vi "Guaman_Estrada_lv_DB_1_II_parcial.vi"() -> ()   [LabVIEW 2014]
panel:
  out "Array":bool[](array[boolean])
  in  "milliseconds to wait 2":u32
  in  "Boolean":bool
  in  "stop":bool
  in  "milliseconds to wait":u32
  out "led 8":bool
  out "led 7":bool
  out "led 6":bool
  out "led 5":bool
  out "led 4":bool
  out "led 3":bool
  out "led_ 2":bool
  out "led_1":bool
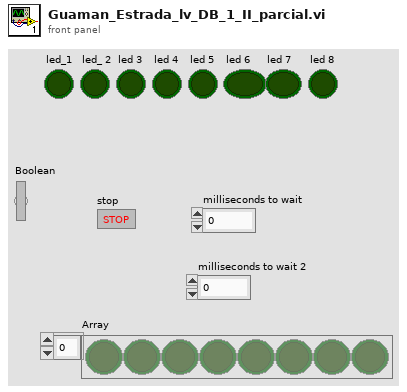
[diagram p1: front panel]
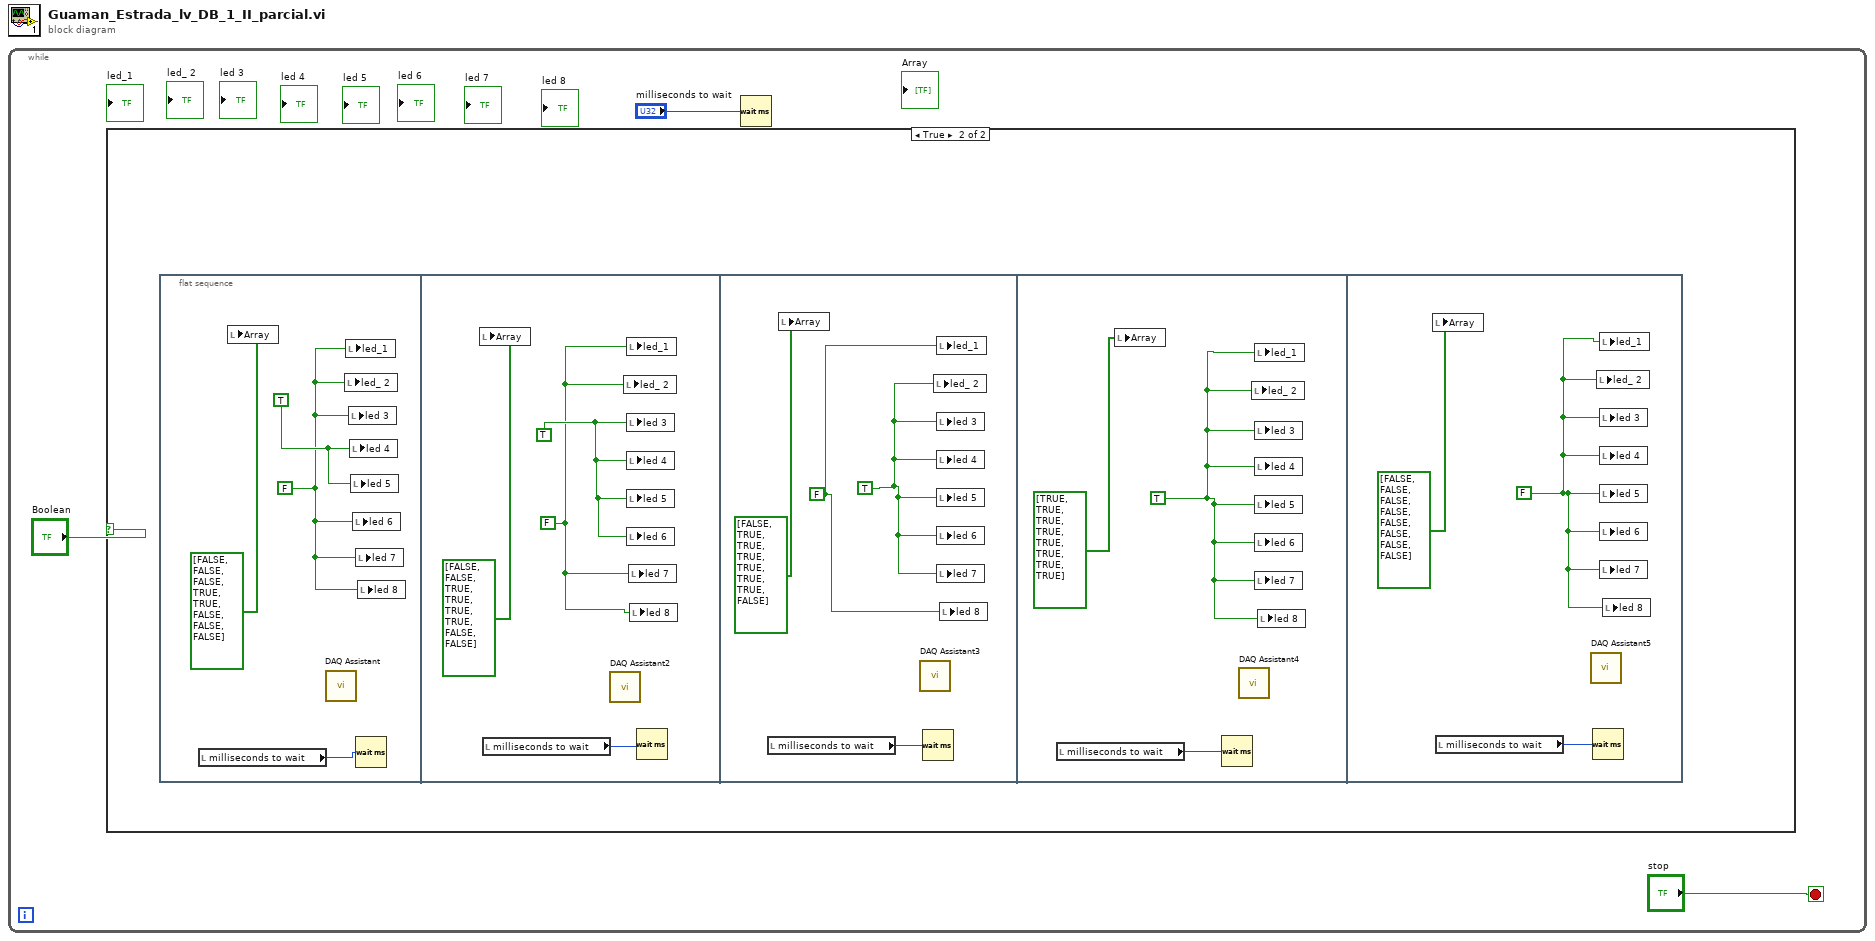
[diagram p0: block diagram]
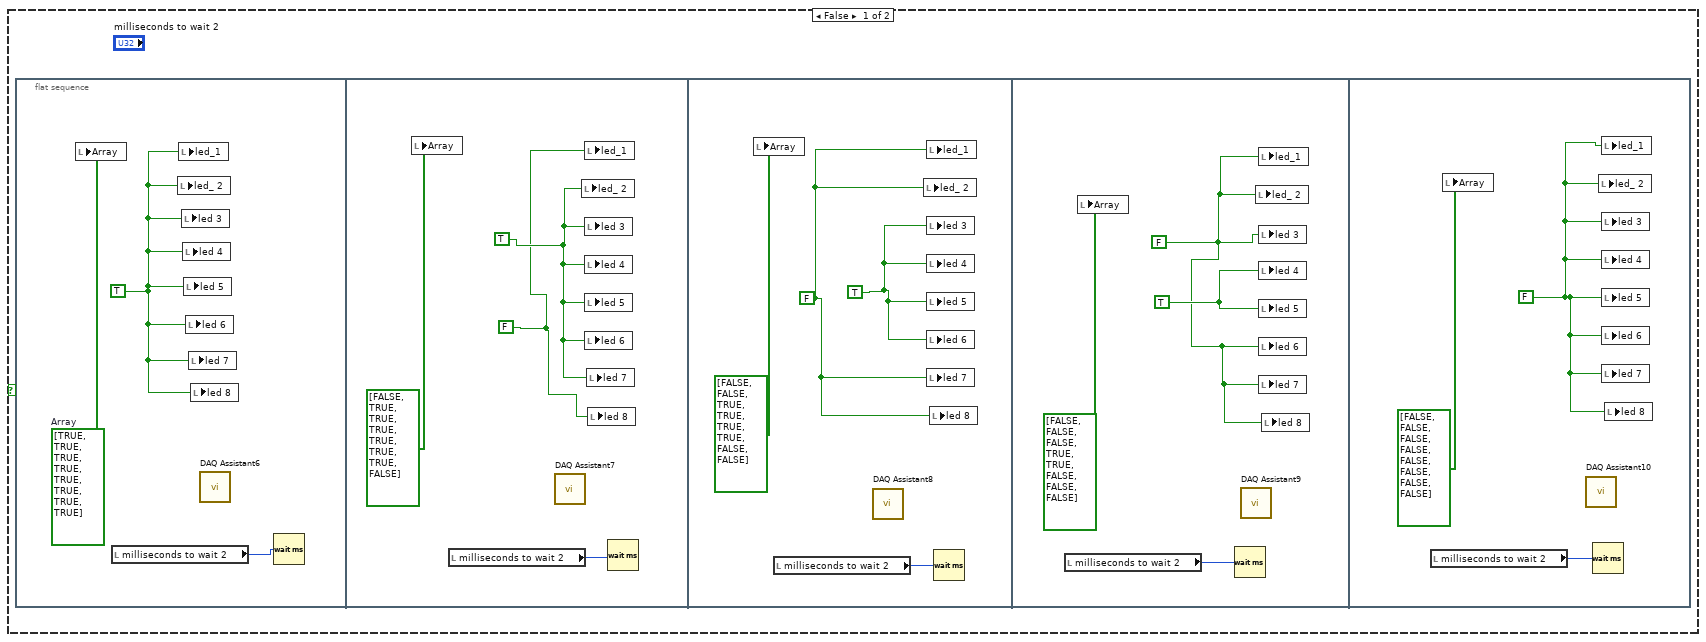
[diagram p2: hidden frame]
diagram:
  n1 = while {
    stop <- "stop" stop-if-true
    n2 = case shown="True" "Boolean" {
      frame False {
        n3 = flat-sequence {
          frame #0 {
            w4 = bool[] [TRUE, TRUE, TRUE, TRUE, TRUE, TRUE, TRUE, TRUE]  # Array
            w5 = TRUE ("led_1")
            n4 = local write "Array"(w4) -> ()
            n5 = local read "milliseconds to wait 2"() -> (w6:u32)
            n6 = local write "led_ 2"(w5) -> ()
            n7 = local write "led_1"(w5) -> ()
            n8 = local write "led 3"(w5) -> ()
            n9 = local write "led 4"(w5) -> ()
            n10 = local write "led 5"(w5) -> ()
            n11 = local write "led 6"(w5) -> ()
            n12 = local write "led 7"(w5) -> ()
            n13 = local write "led 8"(w5) -> ()
            n14 = call "DAQ Assistant6"() -> ()  [unwired: 12 in]
            n15 = Wait (ms)(milliseconds to wait=w6) -> ()  [unwired: 1 out]
          }
          frame #1 {
            w8 = FALSE ("led_1")
            w9 = TRUE ("led_1")
            n16 = local write "Array"(bool[] [FALSE, TRUE, TRUE, TRUE, TRUE, TRUE, TRUE, FALSE] ("Array")) -> ()
            n17 = local read "milliseconds to wait 2"() -> (w10:u32)
            n18 = call "DAQ Assistant7"() -> ()  [unwired: 12 in]
            n19 = local write "led_ 2"(w9) -> ()
            n20 = local write "led_1"(w8) -> ()
            n21 = local write "led 3"(w9) -> ()
            n22 = local write "led 4"(w9) -> ()
            n23 = local write "led 5"(w9) -> ()
            n24 = local write "led 6"(w9) -> ()
            n25 = local write "led 7"(w9) -> ()
            n26 = local write "led 8"(w8) -> ()
            n27 = Wait (ms)(milliseconds to wait=w10) -> ()  [unwired: 1 out]
          }
          frame #2 {
            w12 = FALSE ("led_1")
            w14 = TRUE ("led_1")
            n28 = local write "Array"(bool[] [FALSE, FALSE, TRUE, TRUE, TRUE, TRUE, FALSE, FALSE] ("Array")) -> ()
            n29 = local read "milliseconds to wait 2"() -> (w13:u32)
            n30 = call "DAQ Assistant8"() -> ()  [unwired: 12 in]
            n31 = local write "led_ 2"(w12) -> ()
            n32 = local write "led_1"(w12) -> ()
            n33 = local write "led 3"(w14) -> ()
            n34 = local write "led 4"(w14) -> ()
            n35 = local write "led 5"(w14) -> ()
            n36 = local write "led 6"(w14) -> ()
            n37 = local write "led 7"(w12) -> ()
            n38 = local write "led 8"(w12) -> ()
            n39 = Wait (ms)(milliseconds to wait=w13) -> ()  [unwired: 1 out]
          }
          frame #3 {
            w16 = FALSE ("led_1")
            w17 = TRUE ("led_1")
            n40 = local read "milliseconds to wait 2"() -> (w18:u32)
            n41 = local write "Array"(bool[] [FALSE, FALSE, FALSE, TRUE, TRUE, FALSE, FALSE, FALSE] ("Array")) -> ()
            n42 = Wait (ms)(milliseconds to wait=w18) -> ()  [unwired: 1 out]
            n43 = call "DAQ Assistant9"() -> ()  [unwired: 12 in]
            n44 = local write "led_ 2"(w16) -> ()
            n45 = local write "led_1"(w16) -> ()
            n46 = local write "led 3"(w16) -> ()
            n47 = local write "led 4"(w17) -> ()
            n48 = local write "led 5"(w17) -> ()
            n49 = local write "led 6"(w16) -> ()
            n50 = local write "led 7"(w16) -> ()
            n51 = local write "led 8"(w16) -> ()
          }
          frame #4 {
            w21 = FALSE ("led_1")
            n52 = local read "milliseconds to wait 2"() -> (w20:u32)
            n53 = local write "Array"(bool[] [FALSE, FALSE, FALSE, FALSE, FALSE, FALSE, FALSE, FALSE] ("Array")) -> ()
            n54 = call "DAQ Assistant10"() -> ()  [unwired: 12 in]
            n55 = Wait (ms)(milliseconds to wait=w20) -> ()  [unwired: 1 out]
            n56 = local write "led_ 2"(w21) -> ()
            n57 = local write "led_1"(w21) -> ()
            n58 = local write "led 3"(w21) -> ()
            n59 = local write "led 4"(w21) -> ()
            n60 = local write "led 5"(w21) -> ()
            n61 = local write "led 6"(w21) -> ()
            n62 = local write "led 7"(w21) -> ()
            n63 = local write "led 8"(w21) -> ()
          }
        }
      }
      frame True {
        n64 = flat-sequence {
          frame #0 {
            w24 = FALSE ("led_1")
            w25 = TRUE ("led_1")
            n65 = local read "milliseconds to wait"() -> (w23:u32)
            n66 = local write "Array"(bool[] [FALSE, FALSE, FALSE, TRUE, TRUE, FALSE, FALSE, FALSE] ("Array")) -> ()
            n67 = call "DAQ Assistant"() -> ()  [unwired: 12 in]
            n68 = local write "led_ 2"(w24) -> ()
            n69 = local write "led_1"(w24) -> ()
            n70 = local write "led 3"(w24) -> ()
            n71 = local write "led 4"(w25) -> ()
            n72 = local write "led 5"(w25) -> ()
            n73 = local write "led 6"(w24) -> ()
            n74 = local write "led 7"(w24) -> ()
            n75 = Wait (ms)(milliseconds to wait=w23) -> ()  [unwired: 1 out]
            n76 = local write "led 8"(w24) -> ()
          }
          frame #1 {
            w27 = FALSE ("led_1")
            w29 = TRUE ("led_1")
            n77 = local write "Array"(bool[] [FALSE, FALSE, TRUE, TRUE, TRUE, TRUE, FALSE, FALSE] ("Array")) -> ()
            n78 = local read "milliseconds to wait"() -> (w28:u32)
            n79 = call "DAQ Assistant2"() -> ()  [unwired: 12 in]
            n80 = local write "led_ 2"(w27) -> ()
            n81 = local write "led_1"(w27) -> ()
            n82 = local write "led 3"(w29) -> ()
            n83 = local write "led 4"(w29) -> ()
            n84 = local write "led 5"(w29) -> ()
            n85 = local write "led 6"(w29) -> ()
            n86 = local write "led 7"(w27) -> ()
            n87 = local write "led 8"(w27) -> ()
            n88 = Wait (ms)(milliseconds to wait=w28) -> ()  [unwired: 1 out]
          }
          frame #2 {
            w32 = FALSE ("led_1")
            w33 = TRUE ("led_1")
            n89 = local read "milliseconds to wait"() -> (w31:u32)
            n90 = local write "Array"(bool[] [FALSE, TRUE, TRUE, TRUE, TRUE, TRUE, TRUE, FALSE] ("Array")) -> ()
            n91 = call "DAQ Assistant3"() -> ()  [unwired: 12 in]
            n92 = Wait (ms)(milliseconds to wait=w31) -> ()  [unwired: 1 out]
            n93 = local write "led_ 2"(w33) -> ()
            n94 = local write "led_1"(w32) -> ()
            n95 = local write "led 3"(w33) -> ()
            n96 = local write "led 4"(w33) -> ()
            n97 = local write "led 5"(w33) -> ()
            n98 = local write "led 6"(w33) -> ()
            n99 = local write "led 7"(w33) -> ()
            n100 = local write "led 8"(w32) -> ()
          }
          frame #3 {
            w36 = TRUE ("led_1")
            n101 = local read "milliseconds to wait"() -> (w35:u32)
            n102 = local write "Array"(bool[] [TRUE, TRUE, TRUE, TRUE, TRUE, TRUE, TRUE, TRUE] ("Array")) -> ()
            n103 = Wait (ms)(milliseconds to wait=w35) -> ()  [unwired: 1 out]
            n104 = call "DAQ Assistant4"() -> ()  [unwired: 12 in]
            n105 = local write "led_ 2"(w36) -> ()
            n106 = local write "led_1"(w36) -> ()
            n107 = local write "led 3"(w36) -> ()
            n108 = local write "led 4"(w36) -> ()
            n109 = local write "led 5"(w36) -> ()
            n110 = local write "led 6"(w36) -> ()
            n111 = local write "led 7"(w36) -> ()
            n112 = local write "led 8"(w36) -> ()
          }
          frame #4 {
            w39 = FALSE ("led_1")
            n113 = local write "Array"(bool[] [FALSE, FALSE, FALSE, FALSE, FALSE, FALSE, FALSE, FALSE] ("Array")) -> ()
            n114 = local read "milliseconds to wait"() -> (w38:u32)
            n115 = call "DAQ Assistant5"() -> ()  [unwired: 12 in]
            n116 = Wait (ms)(milliseconds to wait=w38) -> ()  [unwired: 1 out]
            n117 = local write "led_ 2"(w39) -> ()
            n118 = local write "led_1"(w39) -> ()
            n119 = local write "led 3"(w39) -> ()
            n120 = local write "led 4"(w39) -> ()
            n121 = local write "led 5"(w39) -> ()
            n122 = local write "led 6"(w39) -> ()
            n123 = local write "led 7"(w39) -> ()
            n124 = local write "led 8"(w39) -> ()
          }
        }
      }
    }
    n125 = Wait (ms)(milliseconds to wait="milliseconds to wait") -> ()  [unwired: 1 out]
  }
